vi "Set Output Format.vi"(8 "error in (no error)":errorcluster, 9 "alignment (none)":enum16{"None", "Left", "Center", "Right"}(ring), 10 "auto wrap? (F)":bool, 11 "HD44780 in":refnum<class "HD44780.lvclass">) -> (0 "error out":errorcluster, 3 "HD44780 out":refnum<class "HD44780.lvclass">)   [LabVIEW 2017, in "HD44780.lvclass"]
uses:
  HD44780.lvclass
  HD44780.lvclass/HD44780.ctl
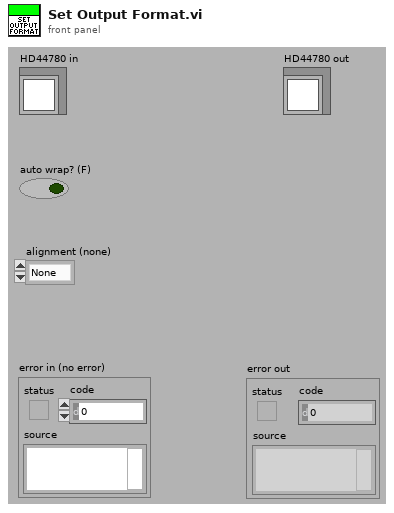
[diagram p1: front panel]
types:
  T1 = typedef "HD44780 Common.lvlib/cluster of class private data.ctl" = cluster{"FPGA VI Reference":refnum<k20>, "device index":i8, "screen size":T2, "font size":T3, "auto wrap":bool, "alignment":T4, "number of line":T5, "shift 0":i8, "entry mode 0":T6, "shift 1":i8, "entry mode 1":T6}
  T2 = typedef "HD44780 Common.lvlib/screen size.ctl" = enum8{"8x1", "8x2", "12x4", "16x1", "16x2", "16x4", "20x1", "20x2", "20x4", "24x1", "24x2", "40x2", "40x4"}
  T3 = typedef "HD44780 Common.lvlib/font size.ctl" = enum8{"5x8", "5x10"}
  T4 = typedef "HD44780 Common.lvlib/alignment.ctl" = enum16{"None", "Left", "Center", "Right"}
  T5 = typedef "HD44780 Common.lvlib/line number.ctl" = enum8{"1 line", "2 lines"}
  T6 = typedef "HD44780 Common.lvlib/entry mode.ctl" = enum8{"increment & no shift", "increment & shift", "decrement & no shift", "decrement & shift"}
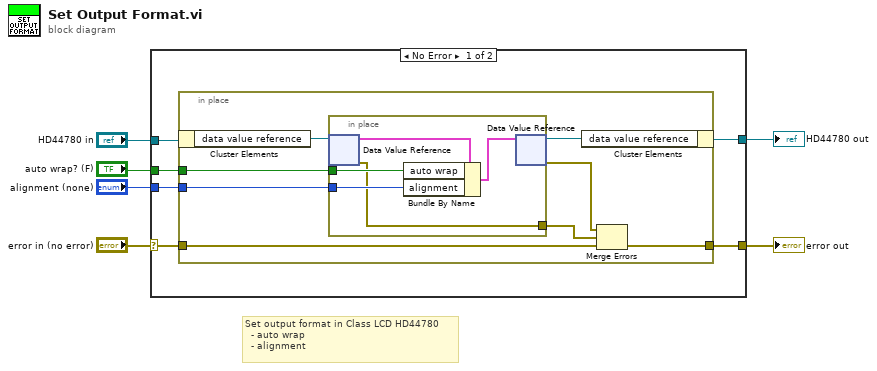
[diagram p0: block diagram]
diagram:
  # "Set output format in Class LCD HD44780\n  - auto wrap\n  - alignment"
  n1 = case shown="No Error" "error in (no error)" {
    selector: "error in (no error)" -> [w8 w27]
    tunnel: [w7 w27] -> w5
    tunnel: [w9 w26] -> w3
    tunnel: "HD44780 in" -> [w10 w26]
    tunnel: "auto wrap? (F)" -> [w12 _]
    tunnel: "alignment (none)" -> [w11 _]
    frame No Error {
      n2 = in-place {
        in-place-border: w12 -> [w20]
        in-place-border: w11 -> [w19]
        in-place-border: w8 -> [w15]
        in-place-border: [w13] -> w7
        n3 = in-place-cluster #1(w10) -> ("data value reference"=w18:refnum<data-value>)
        n4 = in-place {
          in-place-border: w20 -> [w24]
          in-place-border: w19 -> [w23]
          in-place-border: [w21] -> w14
          n5 = in-place-dvr #2(w18) -> (w25:T1, w21:errorcluster)
          n6 = Bundle By Name(cluster=w25, "auto wrap"=w24, "alignment"=w23) -> (w22:T1)
          n7 = in-place-dvr #2(w22) -> (w17:refnum<data-value>, w16:errorcluster)
        }
        n8 = in-place-cluster #1("data value reference"=w17) -> (w9:refnum<class "HD44780.lvclass">)
        n9 = Merge Errors(w16, w14, w15) -> (w13:errorcluster)
      }
    }
    frame Error {
    }
  }
  "error out" <- w5
  "HD44780 out" <- w3
